vi "Filter Cluster Tree_2.vi"(7 "Action":T2=enum."Bundler Insert", 9 "Display Items":T1[](array[typedef]), 10 "Filter Str":string, 11 "Tree Ref":refnum<vi>) -> (0 "error out":errorcluster)   [LabVIEW 2023]
uses:
  controls/action enum.ctl
  cluster/Cluster Element Description.ctl
  utils/Controls/Get-Set Enum.ctl
  Libraries/Tree Handler/Tree Handlr.lvlib
panel:
  out "Filtered Items":T1[](array[typedef])
  in  "C1":T3
  in  "Tree":string[](tree)
  # "DEBUGGARY"
  # "DEBUG"
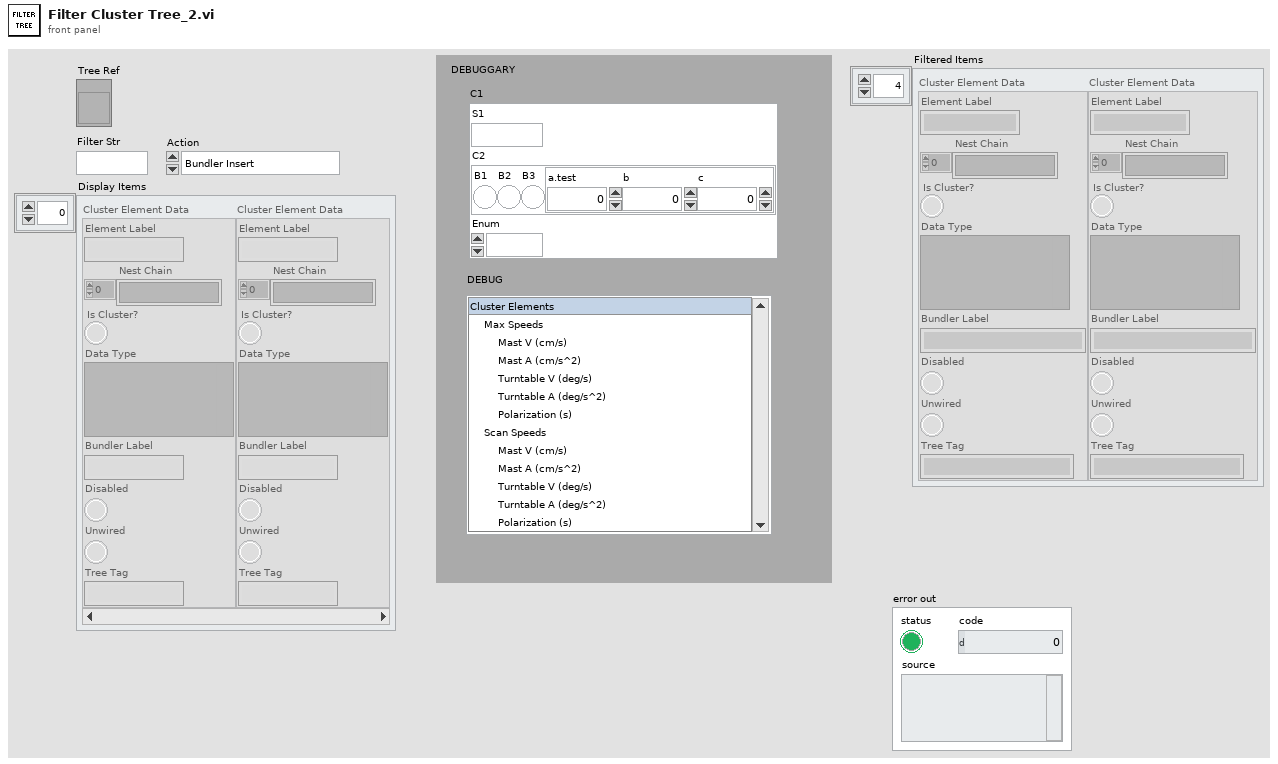
[diagram p1: front panel]
types:
  T1 = typedef "Cluster Element Description.ctl" = cluster{"Element Label":string, "Nest Chain":string[], "Is Cluster?":bool, "Data Type":variant, "Bundler Label":string, "Disabled":bool, "Unwired":bool, "Tree Tag":string}
  T2 = typedef "action enum.ctl" = enum16{"[NONE]", "APP_SEPARATOR", "Wire Bundle", "Wire Unbundle", "Terminal Unbundle", "Terminal Bundle", "Bundler Move Up", "Bundler Move Down", "Bundler Insert", "Bundler Remove", "Bundler Remove Unwired", "Bundler Rearrange", "In Place Insert", "In Place Remove", "In Place Remove Unwired", "In Place Rearrange", "Wire Properties", "Wire Method", "Terminal Properties", "Terminal Method", "Property Move Up", "Property Move Down", "Properties Insert", "Properties Remove", "Properties Remove Unwired", "Properties Rearrange", "Method Change", "Class For Constant", "Class For Control", "Class For Node", "Class Name to Clipboard"}
  T3 = cluster{"S1":string, "C2":cluster{"B1":bool, "B2":bool, "B3":bool, cluster{"a.test":dbl, "b":i32, "c":u8}}, "Enum":enum16{""}}
  T4 = typedef "Get-Set Enum.ctl" = enum16{"Get", "Set"}
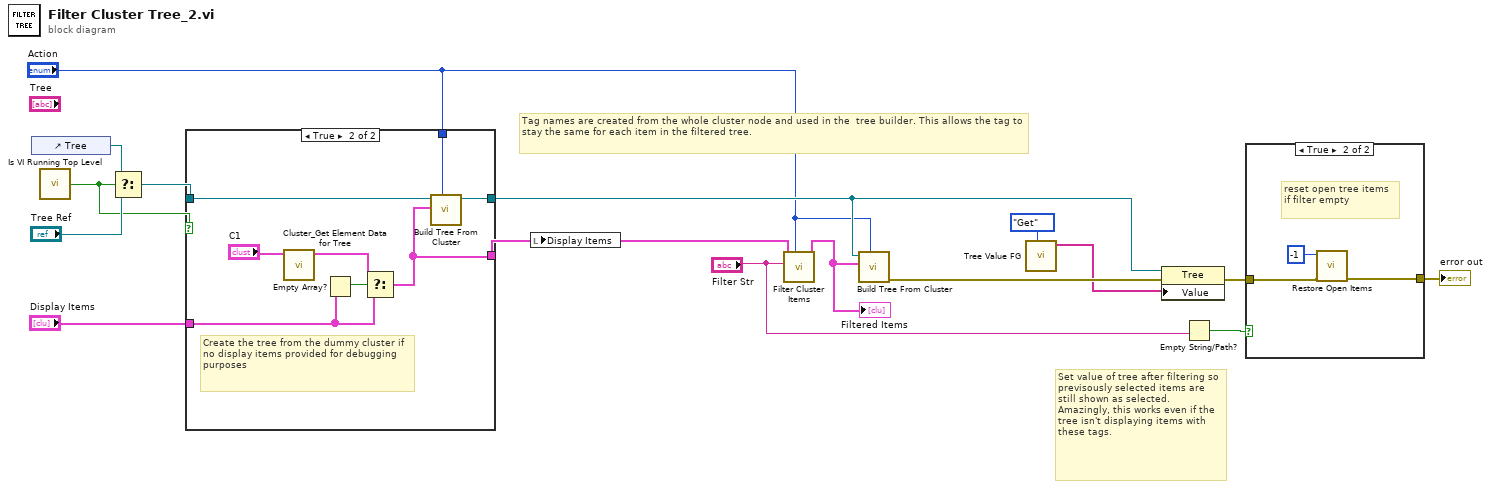
[diagram p0: block diagram]
diagram:
  # "Set value of tree after filtering so previsously selected items are still shown as selected. Amazingly, this works even if the tree isn't displaying items with these tags."
  # "Tag names are created from the whole cluster node and used in the  tree builder. This allows the tag to stay the same for each item in the filtered tree."
  n1 = control-ref of="Tree"() -> (w16:refnum<vi>)
  n2 = call "Is VI Running Top Level.vi"() -> ("Top Level?"=w14:bool)  [unwired: 5 in]
  n3 = Select(t=w16, s=w14, f="Tree Ref") -> (s? t:f=w13:refnum<vi>)
  n4 = case shown="True" w14 {
    tunnel: w13 -> [w18 w26]
    tunnel: [w18 w25] -> w11
    tunnel: [w17 w21] -> w8
    tunnel: "Action" -> [_ w24]
    tunnel: "Display Items" -> [w17 w19]
    frame False {
    }
    frame True {
      # "Create the tree from the dummy cluster if no display items provided for debugging purposes"
      n5 = call "Cluster_Get Element Data for Tree.vi"("Data Type"="C1") -> ("Cluster Element Data Aray"=w22:T1[])  [unwired: 10 in]
      n6 = Empty Array?(array=w19) -> (empty?=w20:bool)
      n7 = Select(t=w22, s=w20, f=w19) -> (s? t:f=w21:T1[])
      n8 = call "Build Tree From Cluster.vi"("Action"=w24, "Display Items"=w21, "Tree Ref"=w26) -> ("Tree Ref Out"=w25:refnum<vi>)  [unwired: 7 in, 1 out]
    }
  }
  n9 = local write "Display Items"(w8) -> ()
  n10 = call "Filter Cluster Items.vi"("Action"="Action", "Filter Str"="Filter Str", "Display Items"=w8) -> ("Filtered Items"=w6:T1[])  [unwired: 8 in]
  "Filtered Items" <- w6
  n11 = call "Build Tree From Cluster.vi"("Action"="Action", "Display Items"=w6, "Tree Ref"=w11) -> ("error out"=w9:errorcluster)  [unwired: 7 in, 1 out]
  n12 = call "Tree Value FG.vi"("Get Set Enum"=Get-Set_Enum."Get") -> ("Compiled Value"=w5:string[])  [unwired: 10 in]
  n13 = property class="Tree"(reference=w11, error in=w9, "Value"=w5) -> (error out=w4:errorcluster)  [unwired: 1 out]
  n14 = Empty String/Path?(string/path="Filter Str") -> (empty?=w2:bool)
  n15 = case shown="True" w2 {
    tunnel: w4 -> [w27 w30]
    tunnel: [w27 w28] -> w3
    frame False {
    }
    frame True {
      # "reset open tree items if filter empty"
      n16 = call "Restore Open Items.vi"("error in"=w30, "Module ID"=-1) -> ("error out"=w28:errorcluster)  [unwired: 9 in]
    }
  }
  "error out" <- w3
